vi "SetTargetPanel.vi"(8 "error in (no error)":errorcluster, 10 "TargetPanel":string, 11 "GRMActor in":refnum<class "GeneralRMActor.lvclass">) -> (0 "error out":errorcluster, 3 "GRMActor out":refnum<class "GeneralRMActor.lvclass">)   [LabVIEW 2020, in "GeneralRMActor.lvlib" / "GeneralRMActor.lvclass"]
uses:
  GeneralRMActor.lvclass
  GeneralRMActor.lvclass/GeneralRMActor.ctl
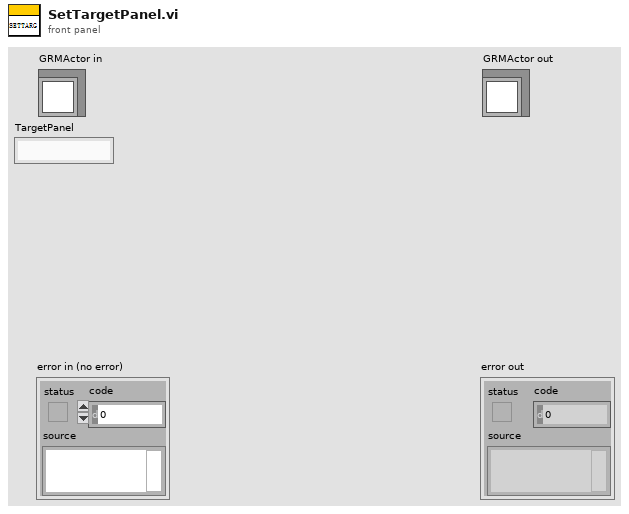
[diagram p1: front panel]
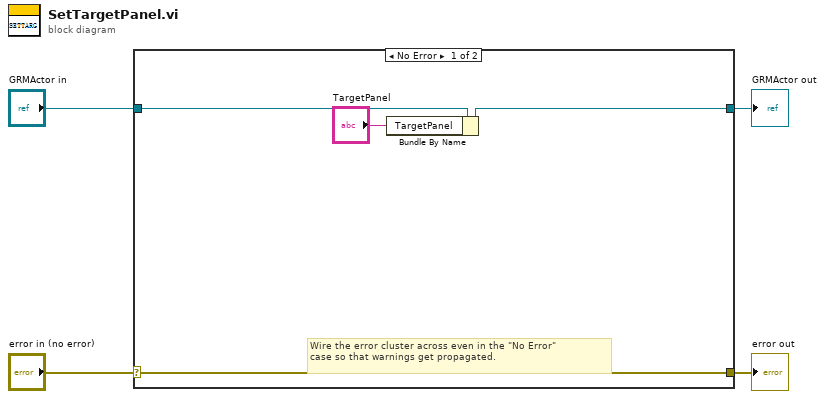
[diagram p0: block diagram]
diagram:
  n1 = case shown="No Error" "error in (no error)" {
    selector: "error in (no error)" -> [w7 w10]
    tunnel: [w7 w10] -> w3
    tunnel: [w6 w9] -> w1
    tunnel: "GRMActor in" -> [w8 w9]
    frame No Error {
      # "Wire the error cluster across even in the \"No Error\"\ncase so that warnings get propagated."
      n2 = Bundle By Name(cluster=w8, "TargetPanel"="TargetPanel") -> (w6:refnum<class "GeneralRMActor.lvclass">)
    }
    frame Error {
    }
  }
  "error out" <- w3
  "GRMActor out" <- w1
